vi "System Subpanel.vi"(11 "CIF_UI in":refnum<class "CIF_UI.lvclass">) -> ()   [LabVIEW 2021, in "CIF Manager UI.lvlib"]
uses:
  CIF Manager UI.lvlib
  CIFUI/Typedef/New Plugin.ctl
  CIFUI/CIF_UI.lvclass
  CIFUI/Typedef/Core UI References.ctl
  CIFUI/CIF_UI.lvclass/CIF_UI.ctl
  CIFUI/UI Element Update/Empty Tree by Reference.vi
  CIFUI/UI Element Update/Empty Table by Reference.vi
  CIFUI/UI Element Update/Initialize Manager Tab by Reference.vi
  CIFUI/Utilities/Get Human Readable Error.vi
  CIFPluginManager/gRPC/CIF_Manager_Client_Wrapper/CIFManagerClientWrapper.lvlib
panel:
  in  "Update Plugin Types":bool
  in  "Load Plugin":bool
  in  "Reset Info":bool
  in  "Get All Info":bool
  in  "Discovered Plugins":string(tree)
  in  "Loaded Plugins":string(tree)
  in  "New Plugin":T1={"Unique Name"="test", "Type"="", "Version (Optional)"=""}
  in  "Abort Plugin":bool
  in  "Plugin to abort":string
  in  "Abort All Plugins":bool
  out "Info":string
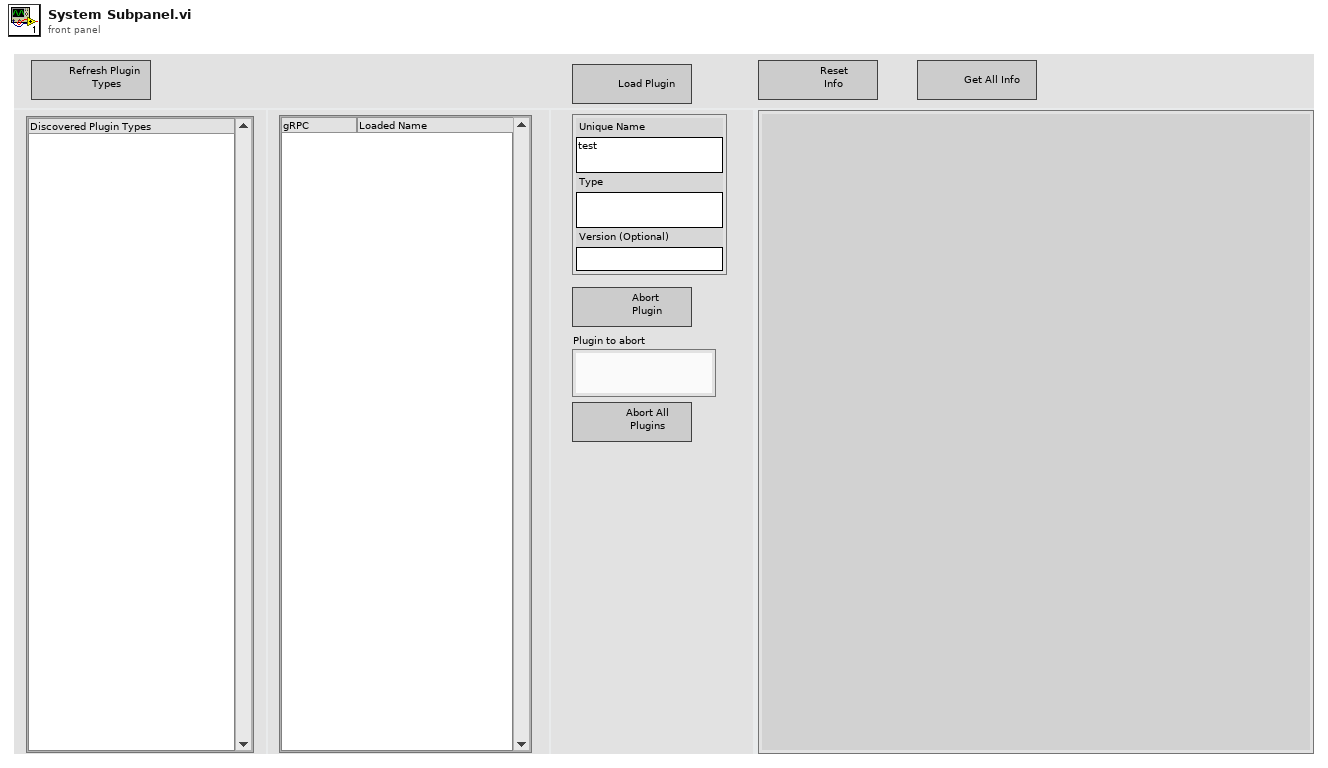
[diagram p1: front panel]
types:
  T1 = typedef "CIF_UI.lvclass/New Plugin.ctl" = cluster{"Unique Name":string, "Type":string, "Version (Optional)":string}
  T2 = typedef "CIF_UI.lvclass/Core UI References.ctl" = cluster{"Discovered Plugins":refnum<vi>, "Discovered Plugins Valid":bool, "Loaded Plugins":refnum<vi>, "Loaded Plugins Valid":bool, "Publisher Channels":refnum<vi>, "Publisher Channels Valid":bool, "Subscriber Channels":refnum<vi>, "Subscriber Channels Valid":bool, "Plugin Status":refnum<vi>, "Plugin Status Valid":bool, "Channel Connection":refnum<vi>, "Channel Connection Valid":bool, "New Plugin Load":refnum<vi>, "New Plugin Load Valid":bool, "Errors":refnum<vi>, "Errors Valid":bool, "Plugin to Abort":refnum<vi>, "Plugin to Abort Valid":bool, "Connection":refnum<vi>, "Connection Valid":bool, "Exit":refnum<vi>, "Exit Valid":bool, "Run Listen":refnum<vi>, "Run Listen Valid":bool, "CIF Manager Tab":refnum<vi>, "Manger Tab Valid":bool, "Clear Local Error":refnum<vi>, "Clear Local Error Valid":bool, "Local Error":refnum<vi>, "Local Error Valid":bool, "System Errors":refnum<vi>, "System Errors Valid":bool}
  T3 = typedef "grpc-lvsupport-release.lvlib/grpcId.ctl" = u64
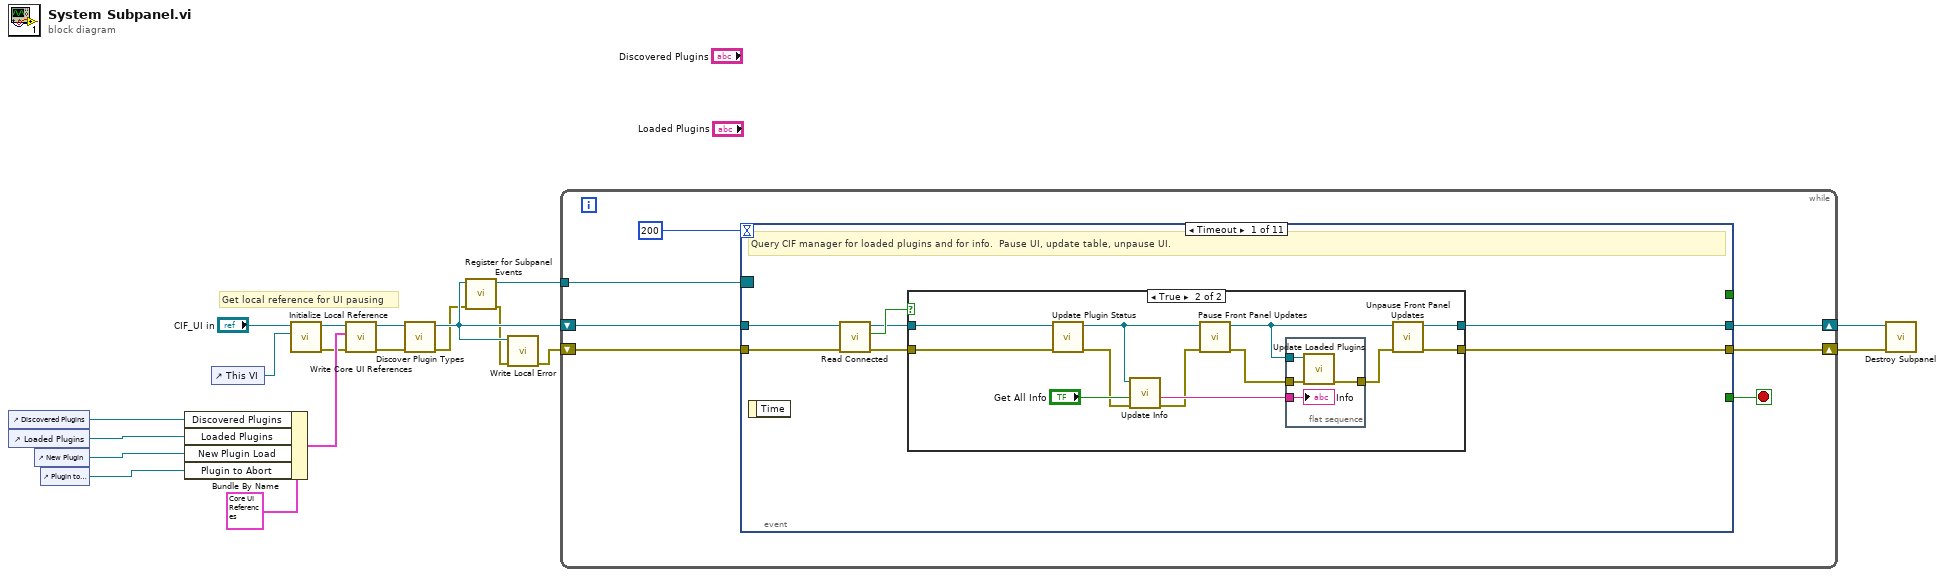
[diagram p0: block diagram]
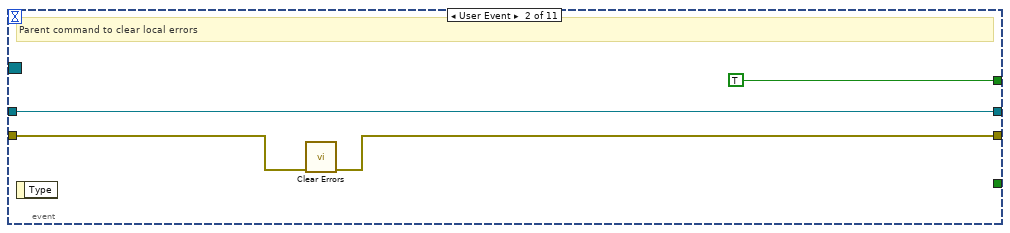
[diagram p3: hidden frame]
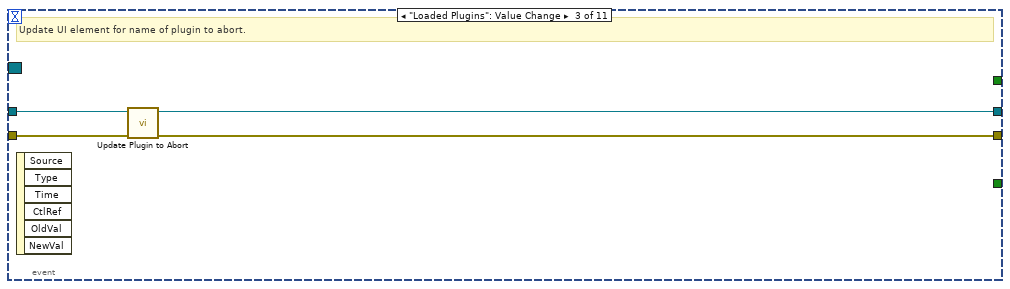
[diagram p4: hidden frame]
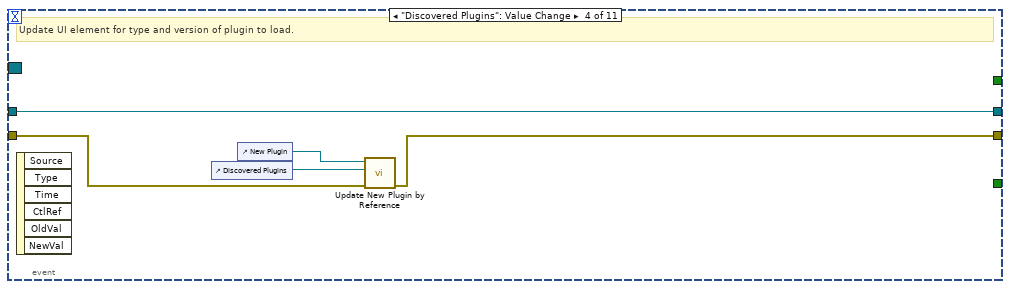
[diagram p5: hidden frame]
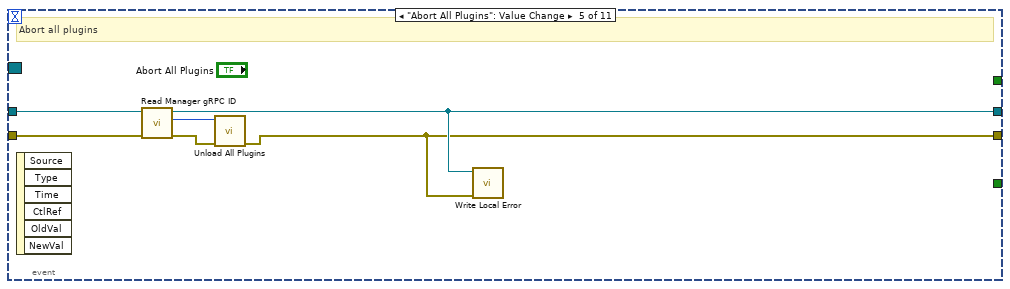
[diagram p6: hidden frame]
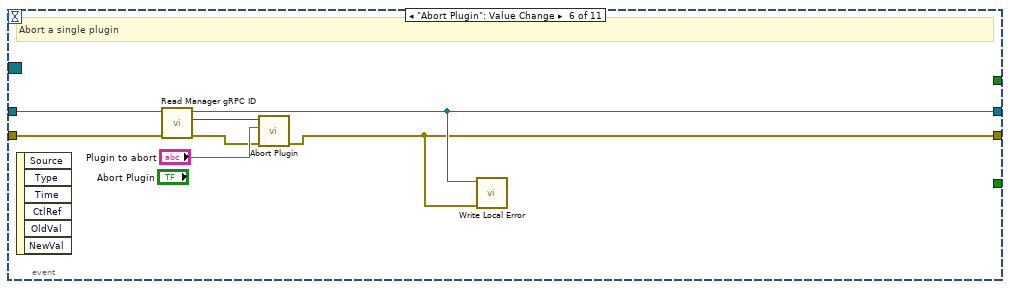
[diagram p7: hidden frame]
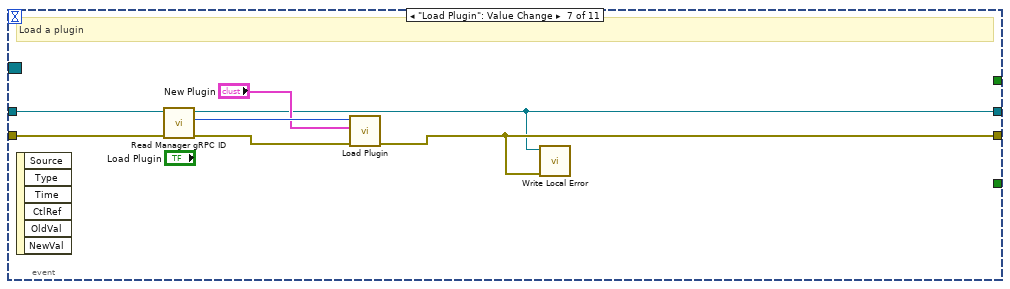
[diagram p8: hidden frame]
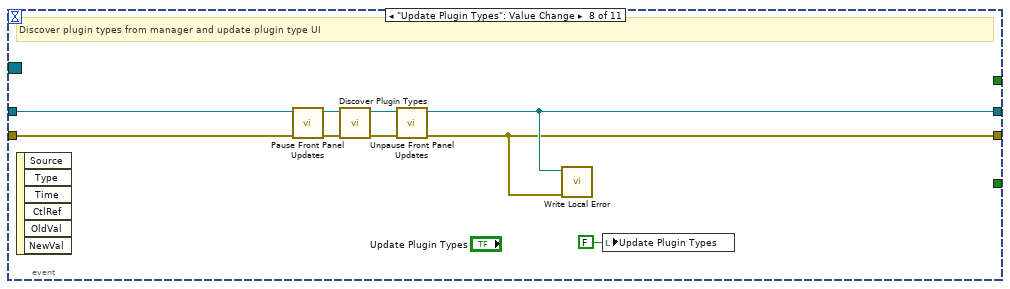
[diagram p9: hidden frame]
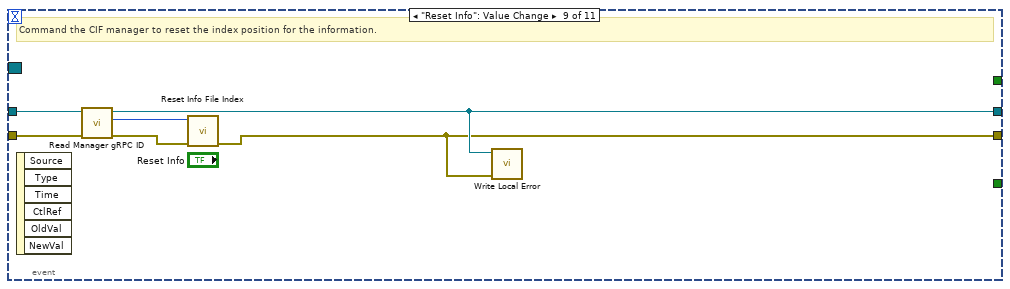
[diagram p10: hidden frame]
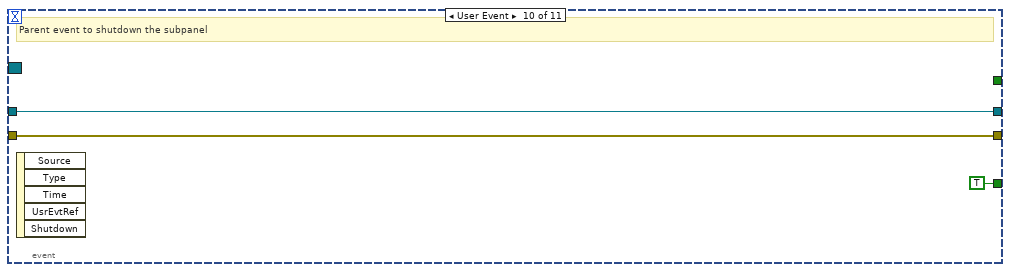
[diagram p11: hidden frame]
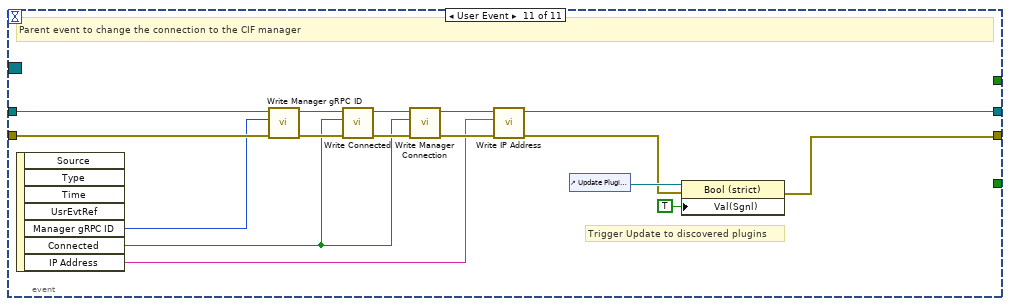
[diagram p12: hidden frame]
diagram:
  # "Get local reference for UI pausing"
  n1 = control-ref of="Discovered Plugins"() -> (w19:refnum<vi>)
  n2 = control-ref of="Loaded Plugins"() -> (w18:refnum<vi>)
  n3 = control-ref of="New Plugin"() -> (w17:refnum<vi>)
  n4 = control-ref of="Plugin to abort"() -> (w16:refnum<vi>)
  n5 = Bundle By Name(cluster=T2 {"Discovered Plugins"=refnum, "Discovered Plugins Valid"=FALSE, "Loaded Plugins"=refnum, "Loaded Plugins Valid"=FALSE, "Publisher Channels"=refnum, "Publisher Channels Valid"=FALSE, "Subscriber Channels"=refnum, "Subscriber Channels Valid"=FALSE, "Plugin Status"=refnum, "Plugin Status Valid"=FALSE, "Channel Connection"=refnum, "Channel Connection Valid"=FALSE, "New Plugin Load"=refnum, "New Plugin Load Valid"=FALSE, "Errors"=refnum, "Errors Valid"=FALSE, "Plugin to Abort"=refnum, "Plugin to Abort Valid"=FALSE, "Connection"=refnum, "Connection Valid"=FALSE, "Exit"=refnum, "Exit Valid"=FALSE, "Run Listen"=refnum, "Run Listen Valid"=FALSE, "CIF Manager Tab"=refnum, "Manger Tab Valid"=FALSE, "Clear Local Error"=refnum, "Clear Local Error Valid"=FALSE, "Local Error"=refnum, "Local Error Valid"=FALSE, "System Errors"=refnum, "System Errors Valid"=FALSE} ("UI References"), "Discovered Plugins"=w19, "Loaded Plugins"=w18, "New Plugin Load"=w17, "Plugin to Abort"=w16) -> (w14:T2)
  n6 = control-ref of="This VI"() -> (w7:refnum<vi>)
  n7 = call "Initialize Local Reference.vi"("This VI"=w7, "CIF_UI in"="CIF_UI in") -> ("error out"=w9:errorcluster, "CIF_UI out"=w10:refnum<class "CIF_UI.lvclass">)  [unwired: 8 in]
  n8 = call "Write Core UI References.vi"("error in (no error)"=w9, "UI References"=w14, "CIF_UI in"=w10) -> ("error out"=w11:errorcluster, "CIF_UI out"=w12:refnum<class "CIF_UI.lvclass">)  [unwired: 7 in]
  n9 = call "Discover Plugin Types.vi"("error in (no error)"=w11, "CIF_UI in"=w12) -> ("error out"=w5:errorcluster, "CIF_UI out"=w6:refnum<class "CIF_UI.lvclass">)  [unwired: 8 in]
  n10 = call "Register for Subpanel Events.vi"("error in (no error)"=w5, "CIF_UI in"=w6) -> ("error out"=w3:errorcluster, "Event Registration Refnum"=w13:refnum<event-registration>)  [unwired: 8 in]
  n11 = call "Write Local Error.vi"("error in (no error)"=w3, "CIF_UI in"=w6) -> ("error out"=w4:errorcluster)  [unwired: 9 in]
  n12 = while {
    shift-right: [w23] -> w2
    shift-left: w6 -> [w22]
    shift-right: [w24] -> w1
    shift-left: w4 -> [w21]
    tunnel: w13 -> [w20]
    stop <- w25 stop-if-true
    n13 = event shown="[0] Timeout" {
      selector: w20 -> [_ _ _ _ _ _ _ _ _ _ _]
      dyn-events: _ -> [_ _ _ _ _ _ _ _ _ _ _]
      timeout: 200 -> [_ _ _ _ _ _ _ _ _ _ _]
      tunnel: [_ _ _ _ _ _ _ _ _ TRUE _] -> w25
      tunnel: w22 -> [w29 w55 w57 w60 w68 w75 w82 w93 w97 w102 w118]
      tunnel: w21 -> [w28 w54 w56 w64 w67 w74 w81 w92 w96 w101 w117]
      tunnel: [w27 w53 w59 w61 w65 w71 w79 w85 w94 w101 w103] -> w24
      tunnel: [w30 w55 w58 w60 w66 w72 w78 w86 w95 w102 w110] -> w23
      tunnel: [_ TRUE _ _ _ _ _ _ _ _ _] -> _
      event Timeout {
        # "Query CIF manager for loaded plugins and for info.  Pause UI, update table, unpause UI."
        n14 = event-data() -> ()  [unwired: 1 in, 1 out]
        n15 = call "Read Connected.vi"("error in (no error)"=w28, "CIF_UI in"=w29) -> ("error out"=w33:errorcluster, "Connected"=w32:bool, "CIF_UI out"=w31:refnum<class "CIF_UI.lvclass">)  [unwired: 7 in]
        n16 = case shown="True" w32 {
          tunnel: w33 -> [w34 w41]
          tunnel: [w34 w47] -> w27
          tunnel: w31 -> [w35 w42]
          tunnel: [w35 w46] -> w30
          frame False {
          }
          frame True {
            n17 = call "Update Plugin Status.vi"("error in (no error)"=w41, "CIF_UI in"=w42) -> ("error out"=w40:errorcluster, "CIF_UI out"=w39:refnum<class "CIF_UI.lvclass">)  [unwired: 8 in]
            n18 = call "Update Info.vi"("error in (no error)"=w40, "Get All Info"="Get All Info", "CIF_UI in"=w39) -> ("error out"=w38:errorcluster, "Info"=w44:string)  [unwired: 7 in]
            n19 = call "Pause Front Panel Updates.vi"("error in (no error)"=w38, "CIF_UI in"=w39) -> ("error out"=w37:errorcluster, "CIF_UI out"=w36:refnum<class "CIF_UI.lvclass">)  [unwired: 8 in]
            n20 = flat-sequence {
              tunnel: w44 -> [w51]
              tunnel: [w50] -> w43
              tunnel: w37 -> [w49]
              tunnel: w36 -> [w48]
              frame #0 {
                n21 = call "Update Loaded Plugins.vi"("error in (no error)"=w49, "CIF_UI in"=w48) -> ("error out"=w50:errorcluster)  [unwired: 9 in]
                "Info" <- w51
              }
            }
            n22 = call "Unpause Front Panel Updates.vi"("error in (no error)"=w43, "CIF_UI in"=w36) -> ("error out"=w47:errorcluster, "CIF_UI out"=w46:refnum<class "CIF_UI.lvclass">)  [unwired: 8 in]
          }
        }
      }
      event User Event {
        # "Parent command to clear local errors"
        n23 = event-data() -> ()  [unwired: 1 in, 1 out]
        n24 = call <vilib>:"Clear Errors.vi"("error in (no error)"=w54) -> ("error out"=w53:errorcluster)  [unwired: 5 in, 1 out]
      }
      event "Loaded Plugins": Value Change {
        # "Update UI element for name of plugin to abort."
        n25 = event-data() -> ()  [unwired: 1 in, 6 out]
        n26 = call "Update Plugin to Abort.vi"("error in (no error)"=w56, "CIF_UI in"=w57) -> ("error out"=w59:errorcluster, "CIF_UI out"=w58:refnum<class "CIF_UI.lvclass">)  [unwired: 8 in]
      }
      event "Discovered Plugins": Value Change {
        # "Update UI element for type and version of plugin to load."
        n27 = event-data() -> ()  [unwired: 1 in, 6 out]
        n28 = control-ref of="Discovered Plugins"() -> (w62:refnum<vi>)
        n29 = control-ref of="New Plugin"() -> (w63:refnum<vi>)
        n30 = call "Update New Plugin by Reference.vi"("error in (no error)"=w64, "Plugin Types Tree"=w62, "New Plugin Control"=w63) -> ("error out"=w61:errorcluster)  [unwired: 8 in]
      }
      event "Abort All Plugins": Value Change {
        # "Abort all plugins"
        n31 = event-data() -> ()  [unwired: 1 in, 6 out]
        n32 = call "Read Manager gRPC ID.vi"("error in (no error)"=w67, "CIF_UI in"=w68) -> ("error out"=w69:errorcluster, "Manager gRPCid"=w70:T3, "CIF_UI out"=w66:refnum<class "CIF_UI.lvclass">)  [unwired: 7 in]
        n33 = call "Unload All Plugins.vi"("error in"=w69, "gRPC ID in"=w70) -> ("error out"=w65:errorcluster)  [unwired: 8 in, 1 out]
        n34 = call "Write Local Error.vi"("error in (no error)"=w65, "CIF_UI in"=w66) -> ()  [unwired: 9 in, 1 out]
      }
      event "Abort Plugin": Value Change {
        # "Abort a single plugin"
        n35 = event-data() -> ()  [unwired: 1 in, 6 out]
        n36 = call "Read Manager gRPC ID.vi"("error in (no error)"=w74, "CIF_UI in"=w75) -> ("error out"=w73:errorcluster, "Manager gRPCid"=w77:T3, "CIF_UI out"=w72:refnum<class "CIF_UI.lvclass">)  [unwired: 7 in]
        n37 = call "Abort Plugin.vi"("error in"=w73, "plugin_name"="Plugin to abort", "gRPC ID in"=w77) -> ("error out"=w71:errorcluster)  [unwired: 7 in, 1 out]
        n38 = call "Write Local Error.vi"("error in (no error)"=w71, "CIF_UI in"=w72) -> ()  [unwired: 9 in, 1 out]
      }
      event "Load Plugin": Value Change {
        # "Load a plugin"
        n39 = event-data() -> ()  [unwired: 1 in, 6 out]
        n40 = call "Read Manager gRPC ID.vi"("error in (no error)"=w81, "CIF_UI in"=w82) -> ("error out"=w83:errorcluster, "Manager gRPCid"=w84:T3, "CIF_UI out"=w78:refnum<class "CIF_UI.lvclass">)  [unwired: 7 in]
        n41 = call "Load Plugin.vi"("error in"=w83, "New Plugin"="New Plugin", "gRPC ID in"=w84) -> ("error out"=w79:errorcluster)  [unwired: 7 in, 1 out]
        n42 = call "Write Local Error.vi"("error in (no error)"=w79, "CIF_UI in"=w78) -> ()  [unwired: 9 in, 1 out]
      }
      event "Update Plugin Types": Value Change {
        # "Discover plugin types from manager and update plugin type UI"
        n43 = event-data() -> ()  [unwired: 1 in, 6 out]
        n44 = call "Pause Front Panel Updates.vi"("error in (no error)"=w92, "CIF_UI in"=w93) -> ("error out"=w91:errorcluster, "CIF_UI out"=w90:refnum<class "CIF_UI.lvclass">)  [unwired: 8 in]
        n45 = call "Discover Plugin Types.vi"("error in (no error)"=w91, "CIF_UI in"=w90) -> ("error out"=w88:errorcluster, "CIF_UI out"=w89:refnum<class "CIF_UI.lvclass">)  [unwired: 8 in]
        n46 = call "Unpause Front Panel Updates.vi"("error in (no error)"=w88, "CIF_UI in"=w89) -> ("error out"=w85:errorcluster, "CIF_UI out"=w86:refnum<class "CIF_UI.lvclass">)  [unwired: 8 in]
        n47 = call "Write Local Error.vi"("error in (no error)"=w85, "CIF_UI in"=w86) -> ()  [unwired: 9 in, 1 out]
        n48 = local write "Update Plugin Types"(FALSE ("Update Plugin Types")) -> ()
      }
      event "Reset Info": Value Change {
        # "Command the CIF manager to reset the index position for the information."
        n49 = event-data() -> ()  [unwired: 1 in, 6 out]
        n50 = call "Read Manager gRPC ID.vi"("error in (no error)"=w96, "CIF_UI in"=w97) -> ("error out"=w98:errorcluster, "Manager gRPCid"=w99:T3, "CIF_UI out"=w95:refnum<class "CIF_UI.lvclass">)  [unwired: 7 in]
        n51 = call "Reset Info File Index.vi"("error in"=w98, "gRPC ID in"=w99) -> ("error out"=w94:errorcluster)  [unwired: 8 in, 1 out]
        n52 = call "Write Local Error.vi"("error in (no error)"=w94, "CIF_UI in"=w95) -> ()  [unwired: 9 in, 1 out]
      }
      event User Event {
        # "Parent event to shutdown the subpanel"
        n53 = event-data() -> ()  [unwired: 1 in, 5 out]
      }
      event User Event {
        # "Trigger Update to discovered plugins"
        # "Parent event to change the connection to the CIF manager"
        n54 = event-data() -> ("Manager gRPC ID"=w109:T3, "Connected"=w108:bool, "IP Address"=w107:string)  [unwired: 1 in, 4 out]
        n55 = call "Write Manager gRPC ID.vi"("error in (no error)"=w117, "gRPCid"=w109, "CIF_UI in"=w118) -> ("error out"=w115:errorcluster, "CIF_UI out"=w116:refnum<class "CIF_UI.lvclass">)  [unwired: 7 in]
        n56 = call "Write Connected.vi"("error in (no error)"=w115, "Connected"=w108, "CIF_UI in"=w116) -> ("error out"=w113:errorcluster, "CIF_UI out"=w114:refnum<class "CIF_UI.lvclass">)  [unwired: 7 in]
        n57 = call "Write Manager Connection.vi"("error in (no error)"=w113, "Manager Connection"=w108, "CIF_UI in"=w114) -> ("error out"=w111:errorcluster, "CIF_UI out"=w112:refnum<class "CIF_UI.lvclass">)  [unwired: 7 in]
        n58 = call "Write IP Address.vi"("error in (no error)"=w111, "IP Address"=w107, "CIF_UI in"=w112) -> ("error out"=w104:errorcluster, "CIF_UI out"=w110:refnum<class "CIF_UI.lvclass">)  [unwired: 7 in]
        n59 = control-ref of="Update Plugin Types"() -> (w106:refnum<vi>)
        n60 = property class="Bool (strict)"(reference=w106, error in=w104, "Val(Sgnl)"=TRUE) -> (error out=w103:errorcluster)  [unwired: 1 out]
      }
    }
  }
  n61 = call "Destroy Subpanel.vi"("error in (no error)"=w1, "CIF_UI in"=w2) -> ()  [unwired: 8 in, 2 out]
